vi "Framework_Initialize.vi"(8 "error in (no error)":errorcluster, 11 "AB_DLL in":refnum<class "AB_DLL.lvclass">) -> (0 "error out":errorcluster, 1 "helpTopics":string[](array[string]), 2 "pageTitles":string[](array[string]), 3 "AB_DLL out":refnum<class "AB_DLL.lvclass">, 4 "helpFile":string, 5 "pages":path[](array[path]))   [LabVIEW 2020, in "AB_DLL.lvclass"]
uses:
  <vilib>/AppBuilder/AB_Classes/DLL/AB_DLL.lvclass
  e:/builds/penguin/labview/branches/2020/dev/dist/vi.lib/AppBuilder/AB_Classes/Build/AB_Build.lvclass
  <vilib>/AppBuilder/AB_Classes/Build/AB_Build.lvclass
panel:
  in  "pageTitles_DLL":string[](array[string])=["Information", "Source Files", "Destinations", "Source File Settings", "Advanced", "Additional Exclusions", "Version Information", "Windows Security", "Run-Time Languages", "Pre/Post Build Actions", "Preview"]
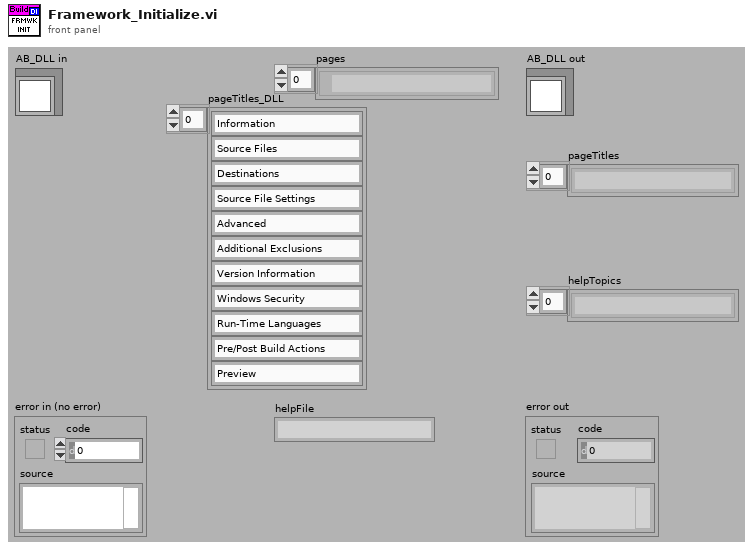
[diagram p1: front panel]
types:
  T1 = enum32{"invalid OS target", "Mac OS", "Windows 3.1", "Windows 95/NT", "Solaris 1", "Solaris 2", "HP-UX", "PowerMAX", "Linux", "Irix", "Rhapsody", "BeOS", "AIX", "OSF1", "VxWorks", "PharLap", "Carbon", "RTX", "Windows x64", "Linux x64", "Mac OS X x64"}
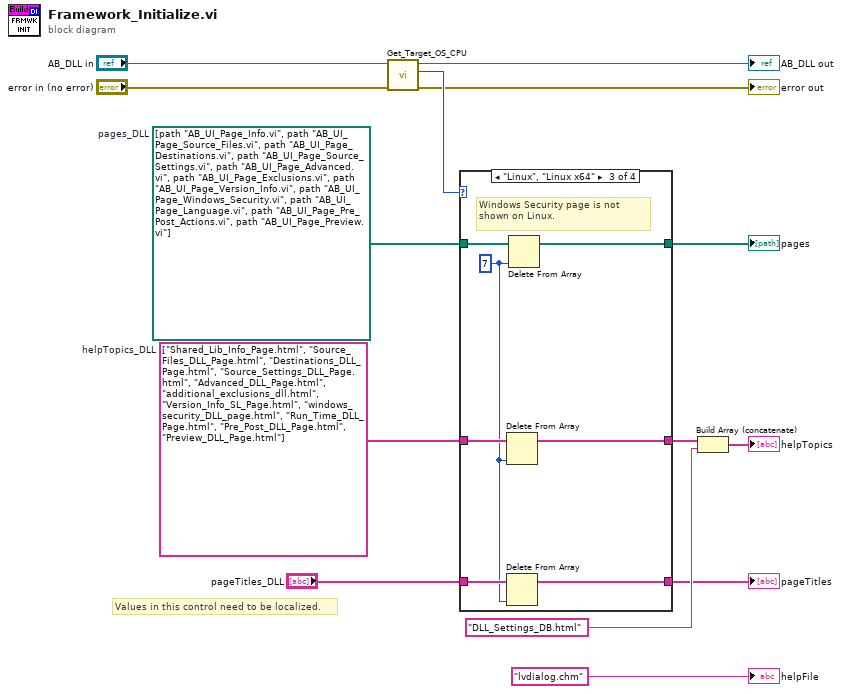
[diagram p0: block diagram]
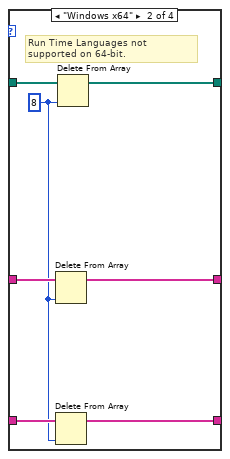
[diagram p3: hidden frame]
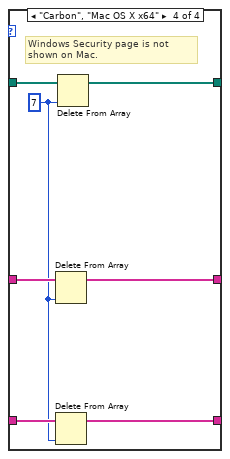
[diagram p4: hidden frame]
diagram:
  w10 = string[] ["Shared_Lib_Info_Page.html", "Source_Files_DLL_Page.html", "Destinations_DLL_Page.html", "Source_Settings_DLL_Page.html", "Advanced_DLL_Page.html", "additional_exclusions_dll.html", "Version_Info_SL_Page.html", "windows_security_DLL_page.html", "Run_Time_DLL_Page.html", "Pre_Post_DLL_Page.html", "Preview_DLL_Page.html"]  # helpTopics_DLL
  w11 = path[] [path "AB_UI_Page_Info.vi", path "AB_UI_Page_Source_Files.vi", path "AB_UI_Page_Destinations.vi", path "AB_UI_Page_Source_Settings.vi", path "AB_UI_Page_Advanced.vi", path "AB_UI_Page_Exclusions.vi", path "AB_UI_Page_Version_Info.vi", path "AB_UI_Page_Windows_Security.vi", path "AB_UI_Page_Language.vi", path "AB_UI_Page_Pre_Post_Actions.vi", path "AB_UI_Page_Preview.vi"]  # pages_DLL
  # "8"
  # "6"
  # "7"
  # "Values in this control need to be localized."
  n1 = call <vilib>:"Get_Target_OS_CPU.vi"("error in (no error)"="error in (no error)", "AB_Build in"="AB_DLL in") -> ("error out"=→"error out":errorcluster, "Target Operating System"=w3:T1, "AB_Build out"=→"AB_DLL out":refnum<class "AB_DLL.lvclass">)  [unwired: 6 in, 1 out]
  n2 = case shown="\"Linux\", \"Linux x64\"" w3 {
    tunnel: w11 -> [w17 w24 w31 w38]
    tunnel: [w17 w20 w27 w34] -> w8
    tunnel: w10 -> [w16 w23 w30 w37]
    tunnel: [w16 w19 w26 w33] -> w9
    tunnel: "pageTitles_DLL" -> [w15 w22 w29 w36]
    tunnel: [w15 w18 w25 w32] -> w6
    frame Default {
    }
    frame "Windows x64" {
      w21 = 8 ("index")
      # "Run Time Languages not supported on 64-bit."
      n3 = Delete From Array(array=w23, index=w21) -> (array with subset deleted=w19:string[])  [unwired: 1 in, 1 out]
      n4 = Delete From Array(array=w22, index=w21) -> (array with subset deleted=w18:string[])  [unwired: 1 in, 1 out]
      n5 = Delete From Array(array=w24, index=w21) -> (array with subset deleted=w20:path[])  [unwired: 1 in, 1 out]
    }
    frame "Linux", "Linux x64" {
      w28 = 7 ("index")
      # "Windows Security page is not shown on Linux."
      n6 = Delete From Array(array=w30, index=w28) -> (array with subset deleted=w26:string[])  [unwired: 1 in, 1 out]
      n7 = Delete From Array(array=w29, index=w28) -> (array with subset deleted=w25:string[])  [unwired: 1 in, 1 out]
      n8 = Delete From Array(array=w31, index=w28) -> (array with subset deleted=w27:path[])  [unwired: 1 in, 1 out]
    }
    frame "Carbon", "Mac OS X x64" {
      w35 = 7 ("index")
      # "Windows Security page is not shown on Mac."
      n9 = Delete From Array(array=w37, index=w35) -> (array with subset deleted=w33:string[])  [unwired: 1 in, 1 out]
      n10 = Delete From Array(array=w36, index=w35) -> (array with subset deleted=w32:string[])  [unwired: 1 in, 1 out]
      n11 = Delete From Array(array=w38, index=w35) -> (array with subset deleted=w34:path[])  [unwired: 1 in, 1 out]
    }
  }
  "pages" <- w8
  "pageTitles" <- w6
  n12 = Build Array (concatenate)(w9, "DLL_Settings_DB.html" ("HTML filename")) -> (→"helpTopics":string[])
  "helpFile" <- "lvdialog.chm" ("CHM or HLP filename (lvdialog.chm)")
